vi "AuMT8852B Power Control Test Configuration.vi"(5 "Settings":T1={"Low frequency selection"=enum."Use low frequency", "Medium frequency selection"=enum."Use medium frequency", "High frequency selection"=enum."Use high frequency", "Low TX frequency"=2402.0, "Low RX frequency"=2480.0, "Medium TX frequency"=2441.0, "Medium RX frequency"=2402.0, "High TX frequency"=2480.0, "High RX frequency"=2402.0, "Number of packets"=1, "Max power step limit"=8.0, "Min power step limit"=2.0, "Packet type"=enum."DH3", "Test control"=enum."Loopback", "Number of cycles"=2, "Minimum power"=-35.0, "Power delay (s)"=1.0} {"Power delay (s)" format="%.2f"; "Minimum power" format="%.2f"; "Min power step limit" format="%.2f"; "Max power step limit" format="%.2f"}, 7 "Set/Get (Set)":enum16{"Set", "Get"}(ring), 8 "error in (no error)":errorcluster, 10 "Script (3)":i32=3, 11 "VISA session":refnum<visa-resource-name>) -> (0 "error out":errorcluster, 2 "error code":i32, 3 "VISA session out":refnum<visa-resource-name>, 4 "Settings out":T1={"Low frequency selection"=enum."Use low frequency", "Medium frequency selection"=enum."Use medium frequency", "High frequency selection"=enum."Use high frequency", "Low TX frequency"=0.0, "Low RX frequency"=0.0, "Medium TX frequency"=0.0, "Medium RX frequency"=0.0, "High TX frequency"=0.0, "High RX frequency"=0.0, "Number of packets"=0, "Max power step limit"=0.0, "Min power step limit"=0.0, "Packet type"=enum."DH1", "Test control"=enum."Loopback", "Number of cycles"=0, "Minimum power"=-30.0, "Power delay (s)"=1.0} {"Power delay (s)" format="%.2f"; "Minimum power" format="%.2f"; "Min power step limit" format="%.2f"; "Max power step limit" format="%.2f"})   [LabVIEW 2017]
doc: "Anritsu MT8852B Bluetooth Tester\n\nConfigures the instrument for the Power Control test.\n\nINPUTS\nSet/Get - whether the values are being sent to or retrieved from the instrument.\nScript - which of the stored scripts (1-10) will be queried or configured. Scripts 1 and 2 are read-only.\nSettings - parameters of the test to be written.\n\nOUTPUTS\nSettings out - current parameters of the test."
uses:
  <instrlib>/aumt8852B/General/Utilities/MT8850 Test Parameters.ctl
  <instrlib>/aumt8852B/General/Utilities/MT8850 Frequency Units.ctl
panel:
  in  "Case Constant\n(See Context Help)":bool
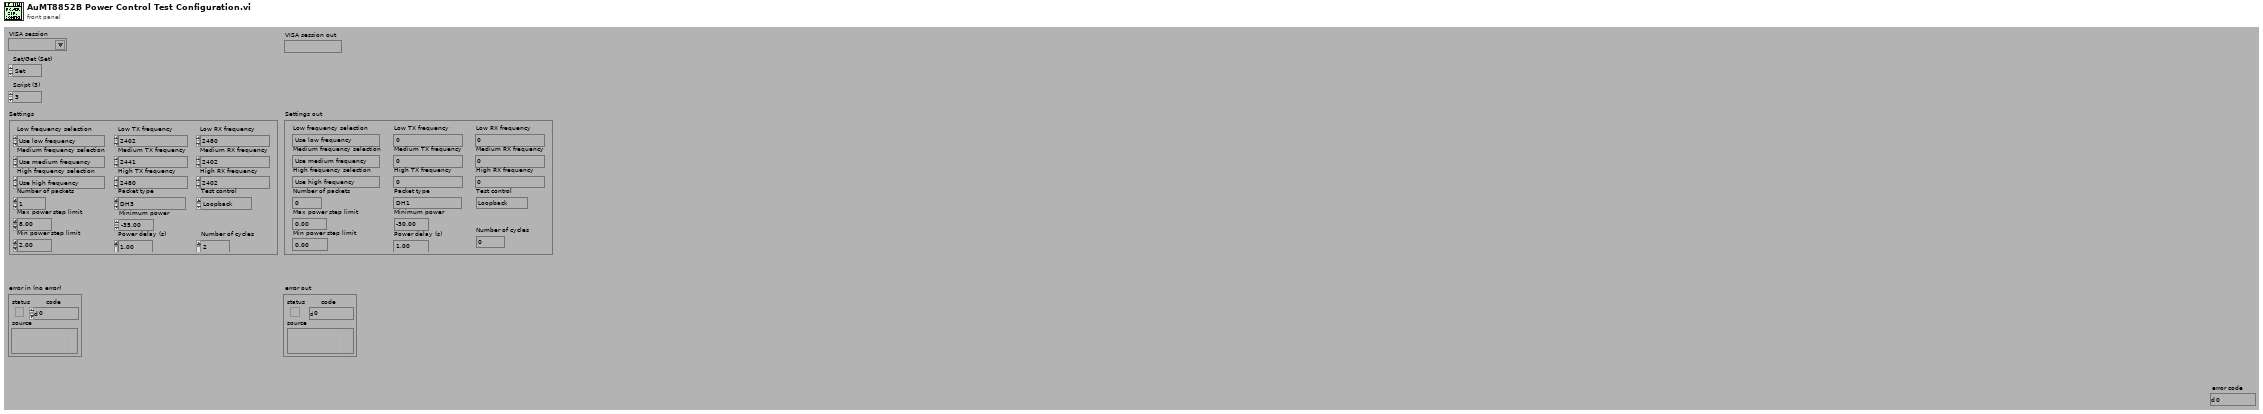
[diagram p1: front panel]
types:
  T1 = cluster{"Low frequency selection":enum16{"Don't use low frequency", "Use low frequency"}, "Medium frequency selection":enum16{"Don't use medium frequency", "Use medium frequency"}, "High frequency selection":enum16{"Don't use high frequency", "Use high frequency"}, "Low TX frequency":dbl, "Low RX frequency":dbl, "Medium TX frequency":dbl, "Medium RX frequency":dbl, "High TX frequency":dbl, "High RX frequency":dbl, "Number of packets":i32, "Max power step limit":dbl, "Min power step limit":dbl, "Packet type":enum16{"DH5", "DH3", "DH1"}, "Test control":enum16{"Loopback", "TX test"}, "Number of cycles":i32, "Minimum power":dbl, "Power delay (s)":dbl}
  T2 = typedef "MT8850 Test Parameters.ctl" = enum16{"Use low frequency", "Use medium frequency", "Use high frequency", "Low TX frequency", "Low RX frquency", "Medium TX frequency", "Medium RX frequency", "High TX frequency", "High RX frequency", "Number of packets", "Average high limit", "Average low limit", "Peak power limit", "Max power step limit", "Min power step limit", "f1 average minimum", "f1 average maximum", "f2 maximum", "f1/f2 average maximum", "Hop selection", "Use DH1 packets", "Use DH3 packets", "Use DH5 packets", "1 slot packet drift limit", "3 slot packet drift limit", "5 slot packet drift limit", "Drift rate limit", "TX power level", "Frequency offset", "Symbol timing", "Modulation index", "BER limit", "FER limit", "Use averaging high limit", "Use averaging low limit", "Use peak power limit", "Packet type", "Test control", "Use max power step limit", "Use min power step limit", "Number of cycles", "Use f1 average maximum", "Use f1 average minimum", "Use f2 maximum", "Use f1/f2 average maximum", "Hop mode", "Maximum negative limit", "Maximum positive limit", "Use maximum negative limit", "Use maximum positive limit", "Use 1 slot packet drift limit", "Use 3 slot packet drift limit", "Use 5 slot packet drift limit", "Use drift rate limit", "Use BER limit", "Use FER limit", "Use dirty parameter table", "Use null packet drift limit", "Null packet drift limit", "Minimum power", "Power delay", "Packet count", "Payload toggle", "Output power level", "2DHX packet type", "3DHX packet type", "Number of blocks", "TX and RX low frequency", "TX and RX medium frequency", "TX and RX high frequency", "TX frequency", "RX frequency", "Threshold bit count", "Total test bit count", "Number of bits", "PDPSK to PGFSK lower limit", "PDPSK to PGFSK upper limit", "Initial frequency error upper limit", "Initial frequency error lower limit", "Frequency error upper limit", "Frequency error lower limit", "Block frequency error upper limit", "Block frequency error lower limit", "2Mbs RMS DEVM limit", "3Mbs RMS DEVM limit", "2Mbs Peak DEVM limit", "3Mbs Peak DEVM limit", "2Mbs 99% packets DEVM limit", "3Mbs 99% packets DEVM limit", "Percentage of no error packets limit", "Threshold error limit", "Total test error limit"}
  T3 = typedef "MT8850 Frequency Units.ctl" = enum16{"Channel", "Hz", "kHz", "MHz", "GHz"}
  T4 = enum16{"Simulate", "Range check", "Cache", "Query instrument status"}
  T5 = enum16{"Output power", "Power control", "Modulation characteristics", "Initial carrier", "Carrier drift", "Single slot sensitivity", "Multiple slot sensitivity", "Maximum input power"}
  T6 = enum16{"Don't use high frequency", "Use high frequency"}
  T7 = enum16{"Don't use medium frequency", "Use medium frequency"}
  T8 = enum16{"Don't use low frequency", "Use low frequency"}
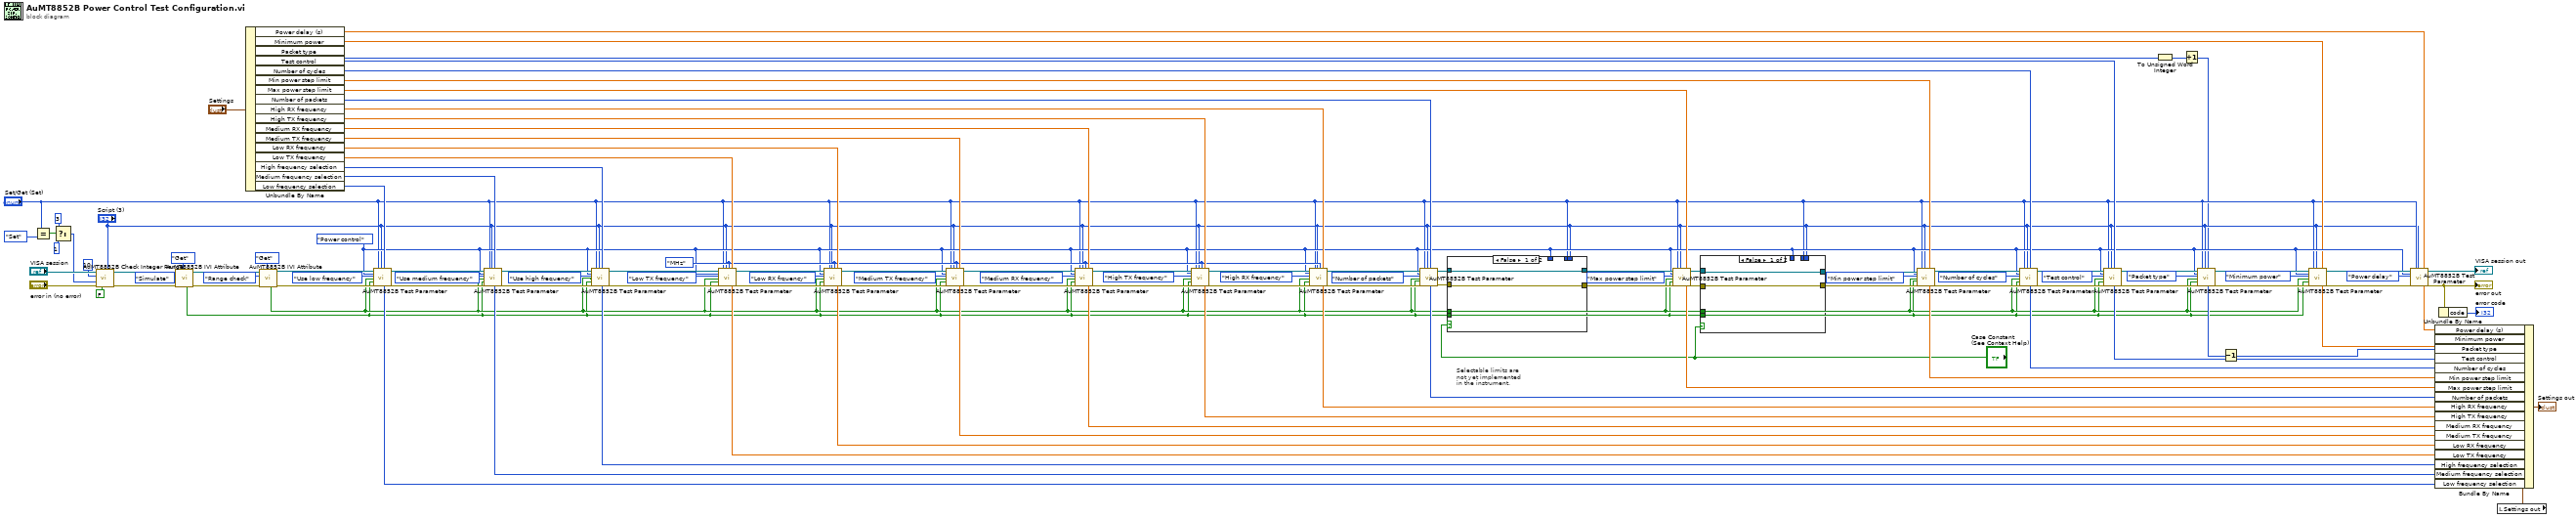
[diagram p0: block diagram]
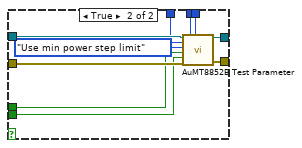
[diagram p2: hidden frame]
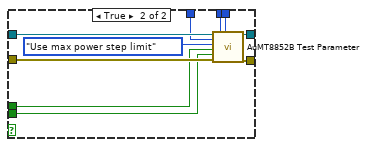
[diagram p3: hidden frame]
diagram:
  w26 = MT8850_Frequency_Units."MHz" ("Frequency units (MHz)")
  w13 = T5."Power control" ("Test (Output Power)")
  # "Selectable limits are\nnot yet implemented\nin the instrument."
  n1 = Equal?(x="Set/Get (Set)", y=enum16{"Set", "Get"}."Set") -> (x = y?=w119:bool)
  n2 = Select(t=3, s=w119, f=1) -> (s? t:f=w115:i32)
  n3 = call <instrlib>:"AuMT8852B Check Integer Range.vi"("Value (0)"="Script (3)", "Check IVI flag first? (T)"=FALSE, "error in (no error)"="error in (no error)", "Lower limit (-1)"=w115, "Upper limit (1)"=10, "VISA session"="VISA session") -> ("error out"=w113:errorcluster, "VISA session out"=w114:refnum<visa-resource-name>)  [unwired: 4 in]
  n4 = call <instrlib>:"AuMT8852B IVI Attribute.vi"("Set/Get (Set)"=enum16{"Set", "Get"}."Get", "error in (no error)"=w113, "Flag (Simulate)"=T4."Simulate", "VISA session"=w114) -> ("error out"=w87:errorcluster, "VISA session out"=w88:refnum<visa-resource-name>, "Value out"=w17:bool)  [unwired: 5 in]
  n5 = Unbundle By Name("Settings") -> ("Power delay (s)"=w6:dbl, "Minimum power"=w7:dbl, "Packet type"=w22:enum16{"DH5", "DH3", "DH1"}, "Test control"=w44:enum16{"Loopback", "TX test"}, "Number of cycles"=w45:i32, "Min power step limit"=w57:dbl, "Max power step limit"=w58:dbl, "Number of packets"=w59:i32, "High RX frequency"=w74:dbl, "High TX frequency"=w75:dbl, "Medium RX frequency"=w60:dbl, "Medium TX frequency"=w76:dbl, "Low RX frequency"=w77:dbl, "Low TX frequency"=w78:dbl, "High frequency selection"=w79:T6, "Medium frequency selection"=w80:T7, "Low frequency selection"=w81:T8)
  n6 = call <instrlib>:"AuMT8852B IVI Attribute.vi"("Set/Get (Set)"=enum16{"Set", "Get"}."Get", "error in (no error)"=w87, "Flag (Simulate)"=T4."Range check", "VISA session"=w88) -> ("error out"=w85:errorcluster, "VISA session out"=w86:refnum<visa-resource-name>, "Value out"=w18:bool)  [unwired: 5 in]
  n7 = call <instrlib>:"AuMT8852B Test Parameter.vi"("VISA session"=w86, "Test (Output power)"=w13, "Parameter (Use low frequency)"=MT8850_Test_Parameters."Use low frequency", "Range check? (F)"=w18, "Simulate? (F)"=w17, "error in (no error)"=w85, "Set/Get (Set)"="Set/Get (Set)", "Script (3)"="Script (3)", "Integer value (0)"=w81) -> ("Integer value out"=w66:i32, "VISA session out"=w33:refnum<visa-resource-name>, "error out"=w32:errorcluster)  [unwired: 7 in, 1 out]
  n8 = call <instrlib>:"AuMT8852B Test Parameter.vi"("VISA session"=w33, "Test (Output power)"=w13, "Parameter (Use low frequency)"=MT8850_Test_Parameters."Use medium frequency", "Range check? (F)"=w18, "Simulate? (F)"=w17, "error in (no error)"=w32, "Set/Get (Set)"="Set/Get (Set)", "Script (3)"="Script (3)", "Integer value (0)"=w80) -> ("Integer value out"=w67:i32, "VISA session out"=w31:refnum<visa-resource-name>, "error out"=w30:errorcluster)  [unwired: 7 in, 1 out]
  n9 = call <instrlib>:"AuMT8852B Test Parameter.vi"("VISA session"=w31, "Test (Output power)"=w13, "Parameter (Use low frequency)"=MT8850_Test_Parameters."Use high frequency", "Range check? (F)"=w18, "Simulate? (F)"=w17, "error in (no error)"=w30, "Set/Get (Set)"="Set/Get (Set)", "Script (3)"="Script (3)", "Integer value (0)"=w79) -> ("Integer value out"=w68:i32, "VISA session out"=w109:refnum<visa-resource-name>, "error out"=w108:errorcluster)  [unwired: 7 in, 1 out]
  n10 = call <instrlib>:"AuMT8852B Test Parameter.vi"("VISA session"=w109, "Test (Output power)"=w13, "Parameter (Use low frequency)"=MT8850_Test_Parameters."Low TX frequency", "Range check? (F)"=w18, "Simulate? (F)"=w17, "error in (no error)"=w108, "Set/Get (Set)"="Set/Get (Set)", "Script (3)"="Script (3)", "Integer value (0)"=w26, "Float value (0)"=w78) -> ("Float value out"=w69:dbl, "VISA session out"=w107:refnum<visa-resource-name>, "error out"=w106:errorcluster)  [unwired: 6 in, 1 out]
  n11 = call <instrlib>:"AuMT8852B Test Parameter.vi"("VISA session"=w107, "Test (Output power)"=w13, "Parameter (Use low frequency)"=MT8850_Test_Parameters."Low RX frquency", "Range check? (F)"=w18, "Simulate? (F)"=w17, "error in (no error)"=w106, "Set/Get (Set)"="Set/Get (Set)", "Script (3)"="Script (3)", "Integer value (0)"=w26, "Float value (0)"=w77) -> ("Float value out"=w70:dbl, "VISA session out"=w105:refnum<visa-resource-name>, "error out"=w104:errorcluster)  [unwired: 6 in, 1 out]
  n12 = call <instrlib>:"AuMT8852B Test Parameter.vi"("VISA session"=w105, "Test (Output power)"=w13, "Parameter (Use low frequency)"=MT8850_Test_Parameters."Medium TX frequency", "Range check? (F)"=w18, "Simulate? (F)"=w17, "error in (no error)"=w104, "Set/Get (Set)"="Set/Get (Set)", "Script (3)"="Script (3)", "Integer value (0)"=w26, "Float value (0)"=w76) -> ("Float value out"=w71:dbl, "VISA session out"=w103:refnum<visa-resource-name>, "error out"=w102:errorcluster)  [unwired: 6 in, 1 out]
  n13 = call <instrlib>:"AuMT8852B Test Parameter.vi"("VISA session"=w103, "Test (Output power)"=w13, "Parameter (Use low frequency)"=MT8850_Test_Parameters."Medium RX frequency", "Range check? (F)"=w18, "Simulate? (F)"=w17, "error in (no error)"=w102, "Set/Get (Set)"="Set/Get (Set)", "Script (3)"="Script (3)", "Integer value (0)"=w26, "Float value (0)"=w60) -> ("Float value out"=w64:dbl, "VISA session out"=w101:refnum<visa-resource-name>, "error out"=w100:errorcluster)  [unwired: 6 in, 1 out]
  n14 = call <instrlib>:"AuMT8852B Test Parameter.vi"("VISA session"=w101, "Test (Output power)"=w13, "Parameter (Use low frequency)"=MT8850_Test_Parameters."High TX frequency", "Range check? (F)"=w18, "Simulate? (F)"=w17, "error in (no error)"=w100, "Set/Get (Set)"="Set/Get (Set)", "Script (3)"="Script (3)", "Integer value (0)"=w26, "Float value (0)"=w75) -> ("Float value out"=w72:dbl, "VISA session out"=w99:refnum<visa-resource-name>, "error out"=w98:errorcluster)  [unwired: 6 in, 1 out]
  n15 = call <instrlib>:"AuMT8852B Test Parameter.vi"("VISA session"=w99, "Test (Output power)"=w13, "Parameter (Use low frequency)"=MT8850_Test_Parameters."High RX frequency", "Range check? (F)"=w18, "Simulate? (F)"=w17, "error in (no error)"=w98, "Set/Get (Set)"="Set/Get (Set)", "Script (3)"="Script (3)", "Integer value (0)"=w26, "Float value (0)"=w74) -> ("Float value out"=w73:dbl, "VISA session out"=w97:refnum<visa-resource-name>, "error out"=w96:errorcluster)  [unwired: 6 in, 1 out]
  n16 = call <instrlib>:"AuMT8852B Test Parameter.vi"("VISA session"=w97, "Test (Output power)"=w13, "Parameter (Use low frequency)"=MT8850_Test_Parameters."Number of packets", "Range check? (F)"=w18, "Simulate? (F)"=w17, "error in (no error)"=w96, "Set/Get (Set)"="Set/Get (Set)", "Script (3)"="Script (3)", "Integer value (0)"=w59) -> ("Integer value out"=w63:i32, "VISA session out"=w38:refnum<visa-resource-name>, "error out"=w39:errorcluster)  [unwired: 7 in, 1 out]
  n17 = case shown="False" "Case Constant\n(See Context Help)" {
    tunnel: w39 -> [w124 w133]
    tunnel: w38 -> [w123 w132]
    tunnel: [w123 w131] -> w37
    tunnel: [w124 w130] -> w36
    tunnel: w18 -> [_ w129]
    tunnel: w17 -> [_ w128]
    tunnel: w13 -> [_ w127]
    tunnel: "Set/Get (Set)" -> [_ w126]
    tunnel: "Script (3)" -> [_ w125]
    frame False {
    }
    frame True {
      n18 = call <instrlib>:"AuMT8852B Test Parameter.vi"("VISA session"=w132, "Test (Output power)"=w127, "Parameter (Use low frequency)"=MT8850_Test_Parameters."Use max power step limit", "Range check? (F)"=w129, "Simulate? (F)"=w128, "error in (no error)"=w133, "Set/Get (Set)"=w126, "Script (3)"=w125) -> ("VISA session out"=w131:refnum<visa-resource-name>, "error out"=w130:errorcluster)  [unwired: 8 in, 2 out]
    }
  }
  n19 = call <instrlib>:"AuMT8852B Test Parameter.vi"("VISA session"=w37, "Test (Output power)"=w13, "Parameter (Use low frequency)"=MT8850_Test_Parameters."Max power step limit", "Range check? (F)"=w18, "Simulate? (F)"=w17, "error in (no error)"=w36, "Set/Get (Set)"="Set/Get (Set)", "Script (3)"="Script (3)", "Float value (0)"=w58) -> ("Float value out"=w62:dbl, "VISA session out"=w40:refnum<visa-resource-name>, "error out"=w43:errorcluster)  [unwired: 7 in, 1 out]
  n20 = case shown="False" "Case Constant\n(See Context Help)" {
    tunnel: w43 -> [w135 w145]
    tunnel: [w135 w144] -> w42
    tunnel: [w136 w143] -> w41
    tunnel: w40 -> [w136 w142]
    tunnel: w18 -> [_ w141]
    tunnel: w17 -> [_ w140]
    tunnel: w13 -> [_ w139]
    tunnel: "Set/Get (Set)" -> [_ w138]
    tunnel: "Script (3)" -> [_ w137]
    frame False {
    }
    frame True {
      n21 = call <instrlib>:"AuMT8852B Test Parameter.vi"("VISA session"=w142, "Test (Output power)"=w139, "Parameter (Use low frequency)"=MT8850_Test_Parameters."Use min power step limit", "Range check? (F)"=w141, "Simulate? (F)"=w140, "error in (no error)"=w145, "Set/Get (Set)"=w138, "Script (3)"=w137) -> ("VISA session out"=w143:refnum<visa-resource-name>, "error out"=w144:errorcluster)  [unwired: 8 in, 2 out]
    }
  }
  n22 = call <instrlib>:"AuMT8852B Test Parameter.vi"("VISA session"=w41, "Test (Output power)"=w13, "Parameter (Use low frequency)"=MT8850_Test_Parameters."Min power step limit", "Range check? (F)"=w18, "Simulate? (F)"=w17, "error in (no error)"=w42, "Set/Get (Set)"="Set/Get (Set)", "Script (3)"="Script (3)", "Float value (0)"=w57) -> ("Float value out"=w61:dbl, "VISA session out"=w50:refnum<visa-resource-name>, "error out"=w51:errorcluster)  [unwired: 7 in, 1 out]
  n23 = call <instrlib>:"AuMT8852B Test Parameter.vi"("VISA session"=w50, "Test (Output power)"=w13, "Parameter (Use low frequency)"=MT8850_Test_Parameters."Number of cycles", "Range check? (F)"=w18, "Simulate? (F)"=w17, "error in (no error)"=w51, "Set/Get (Set)"="Set/Get (Set)", "Script (3)"="Script (3)", "Integer value (0)"=w45) -> ("Integer value out"=w47:i32, "VISA session out"=w48:refnum<visa-resource-name>, "error out"=w49:errorcluster)  [unwired: 7 in, 1 out]
  n24 = call <instrlib>:"AuMT8852B Test Parameter.vi"("VISA session"=w48, "Test (Output power)"=w13, "Parameter (Use low frequency)"=MT8850_Test_Parameters."Test control", "Range check? (F)"=w18, "Simulate? (F)"=w17, "error in (no error)"=w49, "Set/Get (Set)"="Set/Get (Set)", "Script (3)"="Script (3)", "Integer value (0)"=w44) -> ("Integer value out"=w46:i32, "VISA session out"=w24:refnum<visa-resource-name>, "error out"=w25:errorcluster)  [unwired: 7 in, 1 out]
  n25 = To Unsigned Word Integer(number=w22) -> (unsigned 16bit integer=w1:u16)
  n26 = Increment(x=w1) -> (x+1=w3:u16)
  n27 = call <instrlib>:"AuMT8852B Test Parameter.vi"("VISA session"=w24, "Test (Output power)"=w13, "Parameter (Use low frequency)"=MT8850_Test_Parameters."Packet type", "Range check? (F)"=w18, "Simulate? (F)"=w17, "error in (no error)"=w25, "Set/Get (Set)"="Set/Get (Set)", "Script (3)"="Script (3)", "Integer value (0)"=w3) -> ("Integer value out"=w21:i32, "VISA session out"=w20:refnum<visa-resource-name>, "error out"=w19:errorcluster)  [unwired: 7 in, 1 out]
  n28 = Decrement(x=w21) -> (x-1=w2:i32)
  n29 = call <instrlib>:"AuMT8852B Test Parameter.vi"("VISA session"=w20, "Test (Output power)"=w13, "Parameter (Use low frequency)"=MT8850_Test_Parameters."Minimum power", "Range check? (F)"=w18, "Simulate? (F)"=w17, "error in (no error)"=w19, "Set/Get (Set)"="Set/Get (Set)", "Script (3)"="Script (3)", "Float value (0)"=w7) -> ("Float value out"=w9:dbl, "VISA session out"=w15:refnum<visa-resource-name>, "error out"=w14:errorcluster)  [unwired: 7 in, 1 out]
  n30 = call <instrlib>:"AuMT8852B Test Parameter.vi"("VISA session"=w15, "Test (Output power)"=w13, "Parameter (Use low frequency)"=MT8850_Test_Parameters."Power delay", "error in (no error)"=w14, "Set/Get (Set)"="Set/Get (Set)", "Script (3)"="Script (3)", "Float value (0)"=w6) -> ("Float value out"=w8:dbl, "VISA session out"=→"VISA session out":refnum<visa-resource-name>, "error out"=w11:errorcluster)  [unwired: 9 in, 1 out]
  "error out" <- w11
  n31 = Unbundle By Name(w11) -> ("code"=→"error code":i32)
  n32 = local read "Settings out"() -> (w65:T1)
  n33 = Bundle By Name(cluster=w65, "Power delay (s)"=w8, "Minimum power"=w9, "Packet type"=w2, "Test control"=w46, "Number of cycles"=w47, "Min power step limit"=w61, "Max power step limit"=w62, "Number of packets"=w63, "High RX frequency"=w73, "High TX frequency"=w72, "Medium RX frequency"=w64, "Medium TX frequency"=w71, "Low RX frequency"=w70, "Low TX frequency"=w69, "High frequency selection"=w68, "Medium frequency selection"=w67, "Low frequency selection"=w66) -> (→"Settings out":T1)
